vi "Simple Array - Does Not Contain.vi"() -> ()   [LabVIEW 2017, in "Transparent Assertions.Tests.lvlib" / "Assert Collection Contains.lvlib"]
uses:
  Assert Collection Contains.lvlib
  src/Transparent Assertions/Transparent Assertions.lvlib
panel:
  out "error out":errorcluster
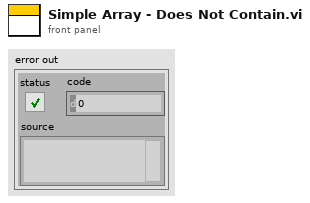
[diagram p1: front panel]
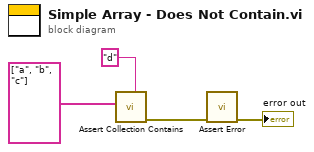
[diagram p0: block diagram]
diagram:
  n1 = call "Assert Collection Contains.vi"("Expected"="d", "Collection"=string[] ["a", "b", "c"]) -> ("error out"=w2:errorcluster)  [unwired: 9 in]
  n2 = call "Assert Error.vi"("error in (no error)"=w2) -> ("error out"=→"error out":errorcluster)  [unwired: 10 in]
